vi "configLVModule.vi"(0 "LV Module":refnum<k7>, 7 "Parameter Indices":i32[](array[numeric]), 9 "Param values":string[](array[string]), 11 "error in":errorcluster, 12 "Default Values":bool[](array[boolean])) -> (15 "error out":errorcluster)   [LabVIEW 2010]
panel:
  out "Numeric":i32
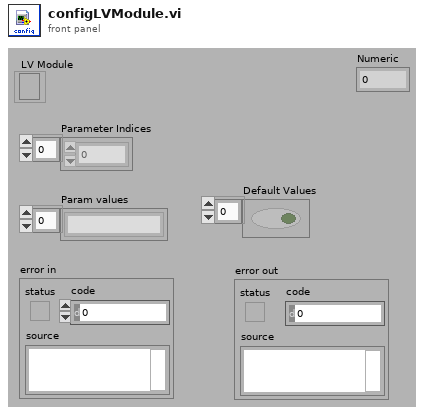
[diagram p1: front panel]
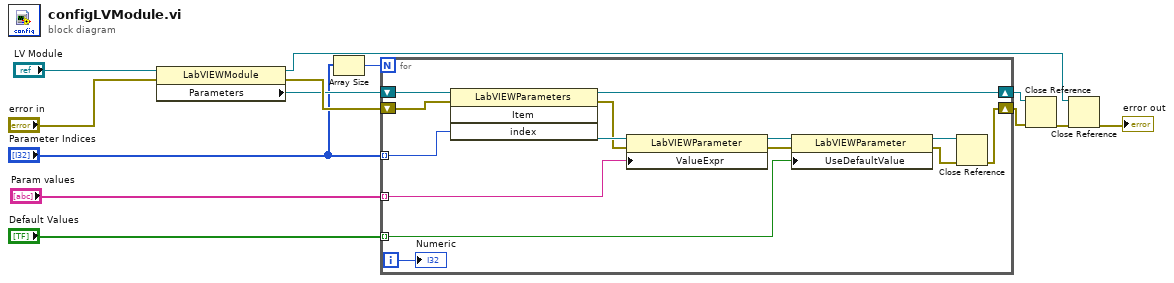
[diagram p0: block diagram]
diagram:
  n1 = property class="LabVIEWModule"(reference="LV Module", error in="error in") -> (reference out=w13:refnum<k7>, error out=w8:errorcluster, "Parameters"=w7:refnum<k7>)
  n2 = Array Size(array="Parameter Indices") -> (size(s)=w2:i32)
  n3 = for {
    N: w2 -> [_]
    tunnel: "Parameter Indices" -> [w25] mode=indexing
    tunnel: "Param values" -> [w22] mode=indexing
    shift-right: [w20] -> w11
    shift-left: w7 -> [w27]
    shift-right: [w21] -> w10
    shift-left: w8 -> [w26]
    tunnel: "Default Values" -> [w15] mode=indexing
    i -> [w14]
    n4 = invoke class="LabVIEWParameters" method="Item"(reference=w27, error in=w26, "index"=w25) -> (reference out=w20:refnum<k7>, error out=w23:errorcluster, "Item"=w24:refnum<k7>)  [unwired: 1 in, 1 out]
    n5 = property class="LabVIEWParameter"(reference=w24, error in=w23, "ValueExpr"=w22) -> (reference out=w19:refnum<k7>, error out=w16:errorcluster)
    n6 = property class="LabVIEWParameter"(reference=w19, error in=w16, "UseDefaultValue"=w15) -> (reference out=w18:refnum<k7>, error out=w17:errorcluster)
    n7 = Close Reference(reference=w18, error in (no error)=w17) -> (error out=w21:errorcluster)
    "Numeric" <- w14
  }
  n8 = Close Reference(reference=w11, error in (no error)=w10) -> (error out=w12:errorcluster)
  n9 = Close Reference(reference=w13, error in (no error)=w12) -> (error out=→"error out":errorcluster)
